vi "ClusterToArray.vi"(8 "error in (no error)":errorcluster, 11 "RingdownConfig":T1={"Config"={"p_SysOdr"=-1, "dThres"=0.0, "Preproc"={"order"=1, "f_lo"=601.0, "f_hi"=10000.0, "R_down"=-1}}, "V index"=0, "I index"=1, "PosSeq"=FALSE}) -> (0 "error out":errorcluster, 3 "RingdownInput":dbl[](array[numeric]))   [LabVIEW 2017, in "AppPlugins.lvlib" / "ERAPlugin.lvclass"]
uses:
  EraPlugin.lvclass
  TypeDef/RingdownConfig.ctl
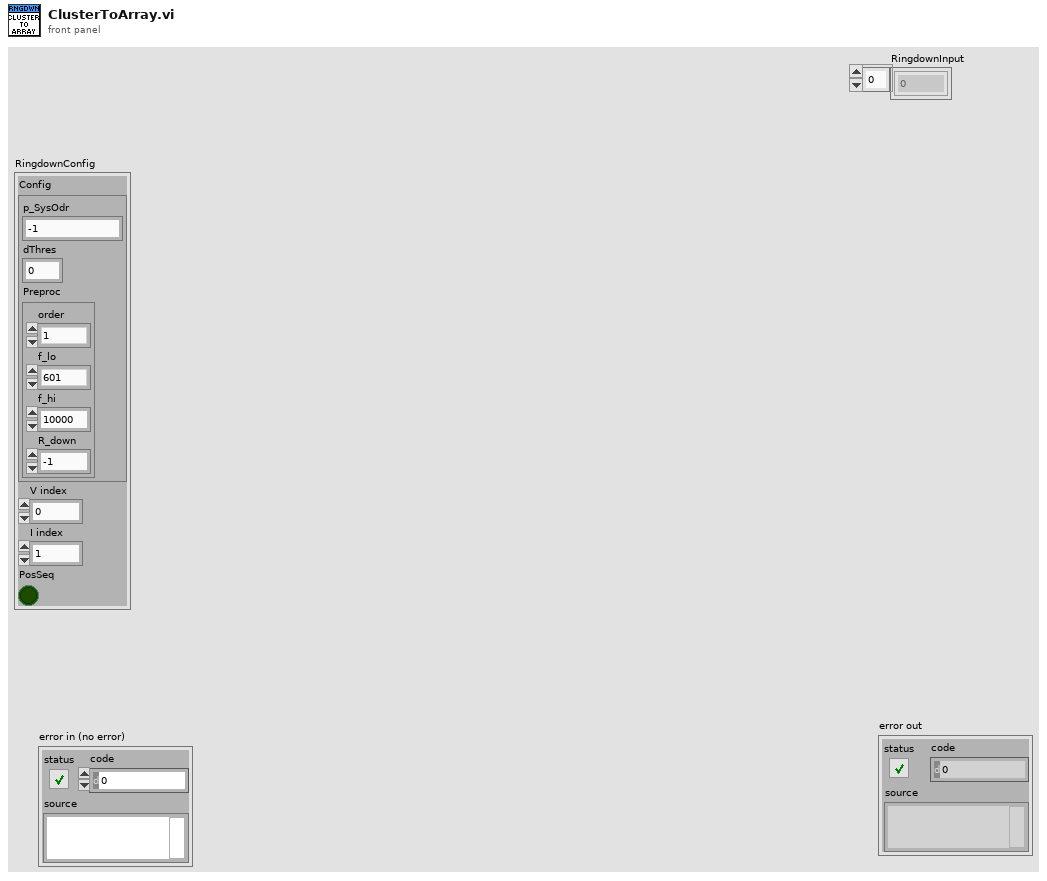
[diagram p1: front panel]
types:
  T1 = typedef "AppPlugins.lvlib/ERAPlugin.lvclass/RingdownConfig.ctl" = cluster{"Config":cluster{"p_SysOdr":i32, "dThres":dbl, "Preproc":cluster{"order":i32, "f_lo":dbl, "f_hi":dbl, "R_down":i32}}, "V index":i32, "I index":i32, "PosSeq":bool}
  T2 = cluster{"p_SysOdr":i32, "dThres":dbl, "Preproc":cluster{"order":i32, "f_lo":dbl, "f_hi":dbl, "R_down":i32}}
  T3 = cluster{"StOffset":i32, "EndOffset":i32, "Length":i32}
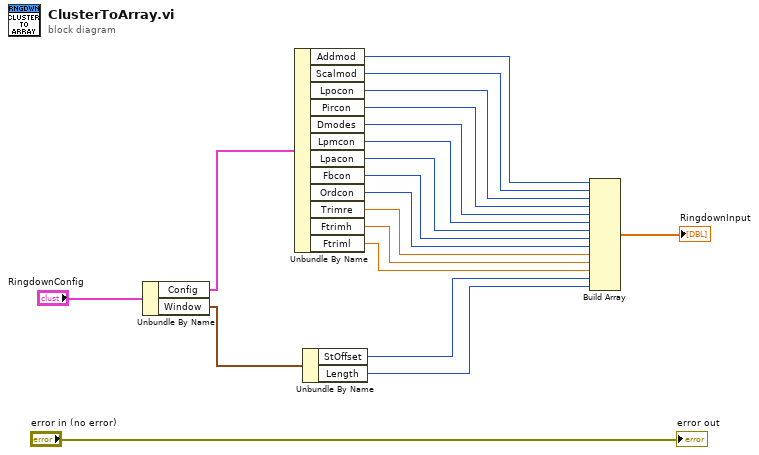
[diagram p0: block diagram]
diagram:
  n1 = Unbundle By Name("RingdownConfig") -> ("Config"=w18:T2, "Window"=w17:T3)
  n2 = Unbundle By Name(w18) -> ("Addmod"=w16:i32, "Scalmod"=w15:i32, "Lpocon"=w14:i32, "Pircon"=w13:i32, "Dmodes"=w12:i32, "Lpmcon"=w11:u16, "Lpacon"=w10:u16, "Fbcon"=w9:u16, "Ordcon"=w8:i32, "Trimre"=w7:dbl, "Ftrimh"=w6:dbl, "Ftriml"=w5:dbl)
  n3 = Unbundle By Name(w17) -> ("StOffset"=w4:i32, "Length"=w3:i32)
  n4 = Build Array(w16, w15, w14, w13, w12, w11, w10, w9, w8, w7, w6, w5, w4, w3) -> (→"RingdownInput":dbl[])
  "error out" <- "error in (no error)"
